vi "RestoreControlValues.vi"(1 "file path":path, 2 "vi path":path) -> (0 "error out":errorcluster)   [LabVIEW 2011]
uses:
  <vilib>/Utility/config.llb/Read Key (String).vi
  <vilib>/Utility/config.llb/NI_LVConfig.lvlib
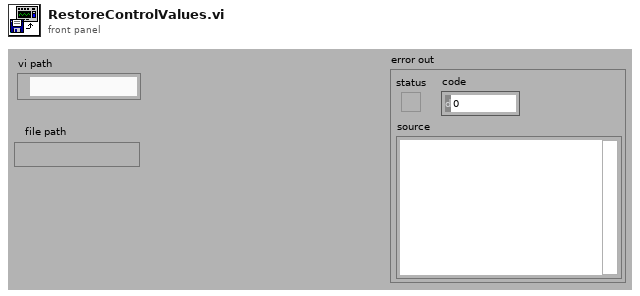
[diagram p1: front panel]
types:
  T1 = typedef "NI_LVConfig.lvlib/Config Data RefNum.ctl" = refnum<k1>
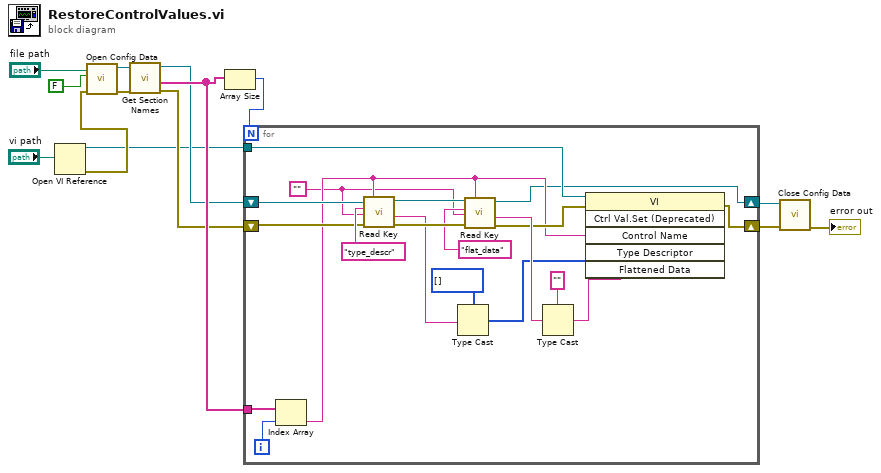
[diagram p0: block diagram]
diagram:
  n1 = Open VI Reference(vi path="vi path") -> (vi reference=w4:refnum<vi>, error out=w5:errorcluster)  [unwired: 5 in]
  n2 = call <vilib>:"Open Config Data.vi"("error in (no error)"=w5, "create file if necessary (T)"=FALSE ("create file if necessary? (T)"), "configuration file path"="file path") -> ("error out"=w10:errorcluster, "refnum"=w11:T1)  [unwired: 6 in, 1 out]
  n3 = call <vilib>:"Get Section Names.vi"("error in (no error)"=w10, "refnum"=w11) -> ("error out"=w6:errorcluster, "section names"=w8:string[], "refnum out"=w7:T1)  [unwired: 7 in]
  n4 = Array Size(array=w8) -> (size(s)=w9:i32)
  n5 = for {
    N: w9 -> [_]
    tunnel: w8 -> [w33]
    shift-right: [w17] -> w1
    shift-left: w7 -> [w30]
    shift-right: [w22] -> w3
    shift-left: w6 -> [w31]
    tunnel: w4 -> [w21]
    i -> [w34]
    w15 = ""
    n6 = Index Array(array=w33, index=w34) -> (element=w19:string)
    n7 = call-poly <vilib>:"Read Key.vi"("section"=w19, "error in (no error)"=w31, "default value"=w15, "key"="type_descr", "refnum"=w30) -> ("error out"=w28:errorcluster, "value"=w27:string, "refnum out"=w29:T1)  [unwired: 3 in, 1 out]
    n8 = Type Cast(type=i16[] [] ("type desc"), x=w27) -> (*(type *) &x=w18:i16[])
    n9 = call-poly <vilib>:"Read Key.vi"("section"=w19, "error in (no error)"=w28, "default value"=w15, "key"="flat_data", "refnum"=w29) -> ("error out"=w23:errorcluster, "value"=w25:string, "refnum out"=w17:T1)  [unwired: 3 in, 1 out]
    n10 = Type Cast(type="" ("flat data"), x=w25) -> (*(type *) &x=w20:string)
    n11 = invoke class="VI" method="Ctrl Val.Set (Deprecated)"(reference=w21, error in=w23, "Control Name"=w19, "Type Descriptor"=w18, "Flattened Data"=w20) -> (error out=w22:errorcluster)  [unwired: 1 in, 5 out]
  }
  n12 = call <vilib>:"Close Config Data.vi"("error in (no error)"=w3, "refnum"=w1) -> ("error out"=→"error out":errorcluster)  [unwired: 8 in, 1 out]
